vi "CH1_ZEROMQ_REP.vi"() -> ()   [LabVIEW 2018]
uses:
  RxTx/CCS_RxTx.lvclass
  <vilib>/addons/zeromq/socket_type.ctl
  <vilib>/addons/zeromq/zmq_socket.lvclass
  <vilib>/addons/zeromq/zmq_context.lvclass
  <vilib>/addons/zeromq/zeromq.lvlib
panel:
  in  "Stop Button":bool
  out "error out 4":errorcluster
  in  "RxTx.lvclass 2":refnum<class "CCS_RxTx.lvclass">
  out "error out 2":errorcluster
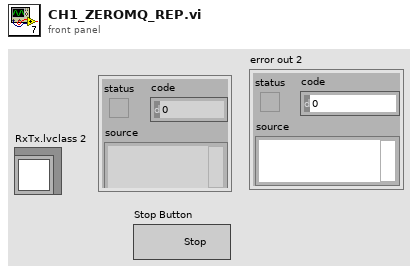
[diagram p1: front panel]
types:
  T1 = typedef "zeromq.lvlib/socket_type.ctl" = enum8{"ZMQ_PAIR", "ZMQ_PUB", "ZMQ_SUB", "ZMQ_REQ", "ZMQ_REP", "ZMQ_DEALER", "ZMQ_ROUTER", "ZMQ_PULL", "ZMQ_PUSH", "ZMQ_XPUB", "ZMQ_XSUB", "ZMQ_STREAM", "ZMQ_SERVER", "ZMQ_CLIENT", "ZMQ_RADIO", "ZMQ_DISH", "ZMQ_GATHER", "ZMQ_SCATTER", "ZMQ_DGRAM"}
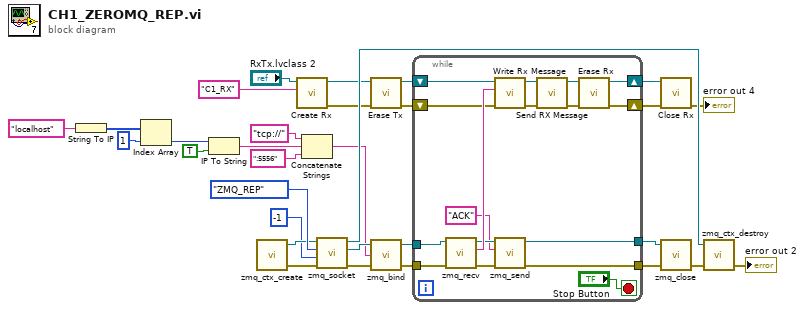
[diagram p0: block diagram]
diagram:
  n1 = String To IP(1:"localhost" ("name")) -> (0:w4:u32[])
  n2 = Index Array(array=w4, index=1) -> (element=w2:u32)
  n3 = IP To String(1:TRUE ("dot notation? (F)"), 2:w2) -> (0:w6:string)
  n4 = call <vilib>:"zmq_ctx_create.vi"() -> ("error out"=w30:errorcluster, "context out"=w29:refnum<class "zmq_context.lvclass">)  [unwired: 4 in]
  n5 = call "Create Rx.vi"("Reader Name"="C1_RX", "RxTx in"="RxTx.lvclass 2") -> ("error out"=w16:errorcluster, "RxTx out"=w17:refnum<class "CCS_RxTx.lvclass">)  [unwired: 8 in]
  n6 = Concatenate Strings("tcp://" ("endpoint"), w6, ":5556" ("endpoint")) -> (w1:string)
  n7 = call <vilib>:"zmq_socket.vi"("error in"=w30, "linger (ms)"=-1, "socket type"=socket_type."ZMQ_REP", "context in"=w29) -> ("error out"=w24:errorcluster, "socket out"=w27:refnum<class "zmq_socket.lvclass">, "context out"=w21:refnum<class "zmq_context.lvclass">)  [unwired: 1 in]
  n8 = call "Erase Tx.vi"("error in (no error)"=w16, "RxTx in"=w17) -> ("error out"=w15:errorcluster, "RxTx out"=w14:refnum<class "CCS_RxTx.lvclass">)  [unwired: 8 in]
  n9 = call <vilib>:"zmq_bind.vi"("error in"=w24, "endpoint"=w1, "socket in"=w27) -> ("error out"=w25:errorcluster, "socket out"=w26:refnum<class "zmq_socket.lvclass">)  [unwired: 1 in]
  n10 = while {
    tunnel: w26 -> [w48]
    tunnel: w25 -> [w47]
    tunnel: [w33] -> w22
    tunnel: [w34] -> w11
    shift-right: [w39] -> w13
    shift-left: w14 -> [w40]
    shift-right: [w38] -> w12
    shift-left: w15 -> [w41]
    stop <- "Stop Button" stop-if-true
    n11 = call <vilib>:"zmq_recv.vi"("error in"=w47, "socket in"=w48) -> ("error out"=w35:errorcluster, "data"=w42:string, "socket out"=w36:refnum<class "zmq_socket.lvclass">)  [unwired: 3 in, 2 out]
    n12 = call "Write Rx Message.vi"("error in (no error)"=w41, "Rx Message"=w42, "RxTx in"=w40) -> ("error out"=w43:errorcluster, "RxTx out"=w44:refnum<class "CCS_RxTx.lvclass">)  [unwired: 7 in]
    n13 = call <vilib>:"zmq_send.vi"("error in"=w35, "data"="ACK", "socket in"=w36) -> ("error out"=w34:errorcluster, "socket out"=w33:refnum<class "zmq_socket.lvclass">)  [unwired: 4 in]
    n14 = call "Send RX Message.vi"("error in (no error)"=w43, "RxTx in"=w44) -> ("error out"=w45:errorcluster, "RxTx out"=w46:refnum<class "CCS_RxTx.lvclass">)  [unwired: 8 in]
    n15 = call "Erase Rx.vi"("error in (no error)"=w45, "RxTx in"=w46) -> ("error out"=w38:errorcluster, "RxTx out"=w39:refnum<class "CCS_RxTx.lvclass">)  [unwired: 8 in]
  }
  n16 = call "Close Rx.vi"("error in (no error)"=w12, "RxTx in"=w13) -> ("error out"=→"error out 4":errorcluster)  [unwired: 8 in, 1 out]
  n17 = call <vilib>:"zmq_close.vi"("error in"=w11, "socket"=w22) -> ("error out"=w23:errorcluster)  [unwired: 3 in]
  n18 = call <vilib>:"zmq_ctx_destroy.vi"("error in"=w23, "context in"=w21) -> ("error out"=→"error out 2":errorcluster)  [unwired: 3 in]
